vi "Read.vi"(8 "error in (no error)":errorcluster, 9 "Sample Rate [Hz]":dbl=1000.0 min=1000.0 max=1000000.0, 10 "Number of Samples":u32=1000, 11 "AI (N Samples) Ref In":T1) -> (0 "error out":errorcluster, 2 "Values":dbl[][](array[numeric]), 3 "AI (N Samples) Ref Out":T1)   [LabVIEW 2021, in "AI Block.lvlib"]
doc: "Reads values from one or more analog input channels. Use this VI to read multiple samples for each channel at one time."
uses:
  <vilib>/myRIO/Instrument Drivers/Onboard IO/AI Block/AI Block.lvlib
  <vilib>/myRIO/Instrument Drivers/Onboard IO/AI Block/typedefs/AI Block Reference.ctl
  <vilib>/myRIO/Common/Instrument Driver Framework/Utilities/typedefs/myRIO Generic Hardware Reference.ctl
  <vilib>/myRIO/Common/Instrument Driver Framework/Utilities/typedefs/Hardware Version Enum.ctl
  <vilib>/myRIO/Common/Instrument Driver Framework/Utilities/typedefs/myRIO v1.0 Reference.ctl
  <vilib>/myRIO/Common/Instrument Driver Framework/Utilities/typedefs/Generic FPGA Reference.ctl
  <vilib>/myRIO/Common/Instrument Driver Framework/myRIO v1.0/AI Block/typedefs/AI Block Channels List.ctl
  <vilib>/myRIO/Common/Instrument Driver Framework/myRIO v1.0/AI Block/typedefs/AI Block Channels Enum.ctl
  <vilib>/myRIO/Common/Instrument Driver Framework/Utilities/typedefs/Analog Scaling Constants.ctl
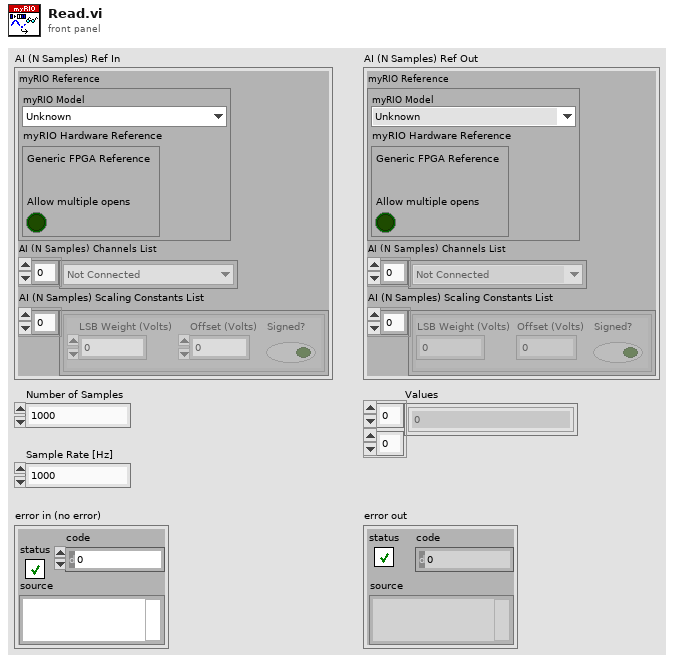
[diagram p1: front panel]
types:
  T1 = typedef "AI Block.lvlib/AI Block Reference.ctl" = cluster{"myRIO Reference":T2, "AI (N Samples) Channels List":T6, "AI (N Samples) Scaling Constants List":T8[]}
  T2 = typedef "myRIO Generic Hardware Reference.ctl" = cluster{"myRIO Model":T3, "myRIO Hardware Reference":T4}
  T3 = typedef "Hardware Version Enum.ctl" = enum16{"Unknown", "myRIO-1900", "myRIO-1950", "roboRIO", "NI ELVIS RIO CM", "ELVIS III"}
  T4 = typedef "myRIO v1.0 Reference.ctl" = cluster{"Generic FPGA Reference":T5, "Allow multiple opens":bool}
  T5 = typedef "Generic FPGA Reference.ctl" = refnum<k20>
  T6 = typedef "AI Block Channels List.ctl" = T7[]
  T7 = typedef "AI Block Channels Enum.ctl" = enum16{"Not Connected", "A/AI0 (N Samples)", "A/AI1 (N Samples)", "A/AI2 (N Samples)", "A/AI3 (N Samples)", "A/AI4 (N Samples)", "A/AI5 (N Samples)", "A/AI6 (N Samples)", "A/AI7 (N Samples)", "A/AI0 (DIFF N Samples)", "A/AI1 (DIFF N Samples)", "A/AI2 (DIFF N Samples)", "A/AI3 (DIFF N Samples)", "B/AI0 (N Samples)", "B/AI1 (N Samples)", "B/AI2 (N Samples)", "B/AI3 (N Samples)", "B/AI4 (N Samples)", "B/AI5 (N Samples)", "B/AI6 (N Samples)", "B/AI7 (N Samples)", "B/AI0 (DIFF N Samples)", "B/AI1 (DIFF N Samples)", "B/AI2 (DIFF N Samples)", "B/AI3 (DIFF N Samples)"}
  T8 = typedef "Analog Scaling Constants.ctl" = cluster{"LSB Weight (Volts)":dbl, "Offset (Volts)":dbl, "Signed?":bool}
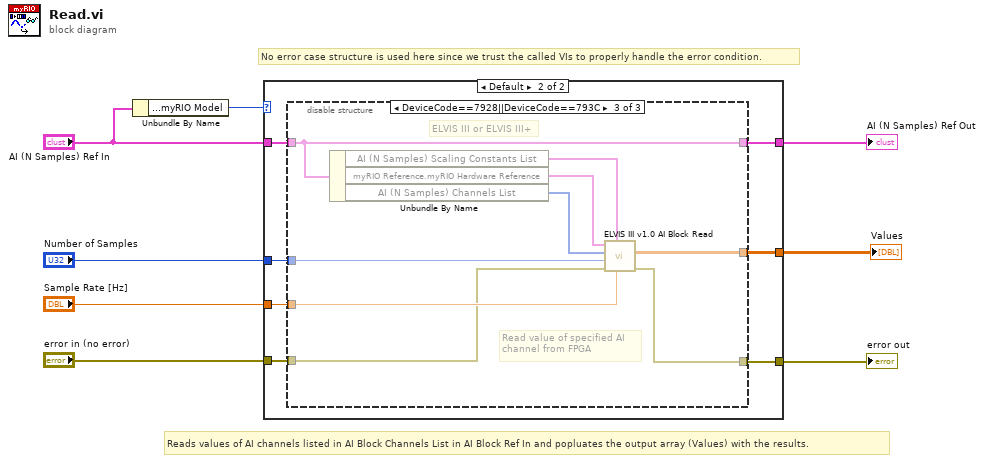
[diagram p0: block diagram]
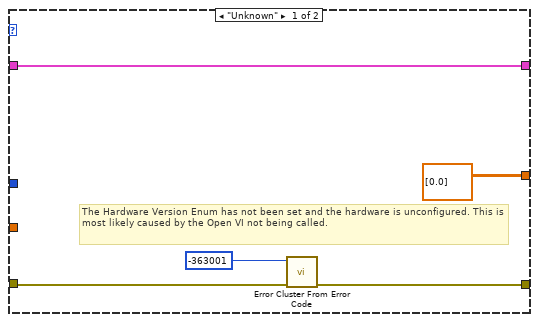
[diagram p2: hidden frame]
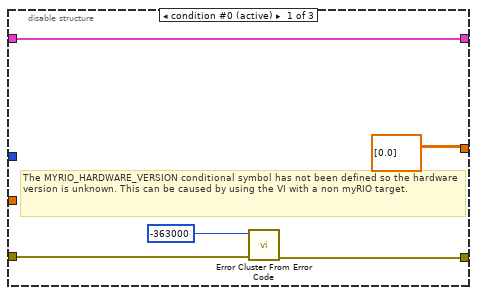
[diagram p3: hidden frame]
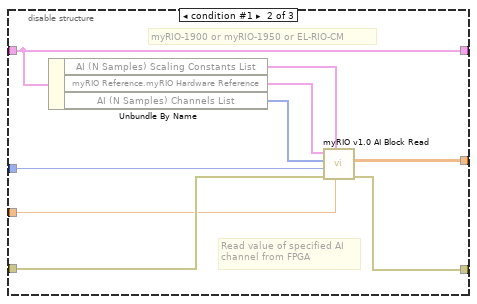
[diagram p4: hidden frame]
diagram:
  # "No error case structure is used here since we trust the called VIs to properly handle the error condition."
  # "Reads values of AI channels listed in AI Block Channels List in AI Block Ref In and popluates the output array (Values) with the results."
  n1 = Unbundle By Name("AI (N Samples) Ref In") -> ("myRIO Reference.myRIO Model"=w3:T3)
  n2 = case shown="Default" w3 {
    tunnel: [w11 w20] -> w5
    tunnel: "AI (N Samples) Ref In" -> [w10 w19]
    tunnel: "error in (no error)" -> [w12 w18]
    tunnel: [w10 w17] -> w6
    tunnel: [dbl[][] [[0.0]] w16] -> w4
    tunnel: "Sample Rate [Hz]" -> [_ w15]
    tunnel: "Number of Samples" -> [_ w14]
    frame "Unknown" {
      # "The Hardware Version Enum has not been set and the hardware is unconfigured. This is most likely caused by the Open VI not being called."
      n3 = call <vilib>:"Error Cluster From Error Code.vi"("error in (no error)"=w12, "error code (0)"=-363001) -> ("error out"=w11:errorcluster)  [unwired: 7 in]
    }
    frame Default {
      n4 = disable-structure shown="DeviceCode==7928||DeviceCode==793C" {
        disable-tunnel: w19 -> [w22 w27 w40]
        disable-tunnel: [w25 w33 w38] -> w20
        disable-tunnel: w18 -> [w23 w34 w35]
        disable-tunnel: [w22 w27 w40] -> w17
        disable-tunnel: [dbl[][] [[0.0]] ("dbl Scaled Value List") w31 w39] -> w16
        disable-tunnel: w15 -> [_ w28 w36]
        disable-tunnel: w14 -> [_ w30 w37]
        frame condition #0 (active) {
          # "The MYRIO_HARDWARE_VERSION conditional symbol has not been defined so the hardware version is unknown. This can be caused by using the VI with a non myRIO target."
          n5 = call <vilib>:"Error Cluster From Error Code.vi"("error in (no error)"=w23, "error code (0)"=-363000) -> ("error out"=w25:errorcluster)  [unwired: 7 in]
        }
        frame condition #1 {
          # "myRIO-1900 or myRIO-1950 or EL-RIO-CM"
          # "Read value of specified AI \nchannel from FPGA"
          n6 = Unbundle By Name(w27) -> ("AI (N Samples) Scaling Constants List"=w26:T8[], "myRIO Reference.myRIO Hardware Reference"=w32:T4, "AI (N Samples) Channels List"=w29:T6)
          n7 = call <vilib>:"myRIO v1.0 AI Block Read.vi"("AI FIFO Sample Rate"=w28, "Scale Constants Array"=w26, "error in (no error)"=w34, "Number of Samples"=w30, "AI (N Samples) Channels List"=w29, "myRIO Ref In"=w32) -> ("error out"=w33:errorcluster, "dbl Scaled Value List"=w31:dbl[][])  [unwired: 3 in, 1 out]
        }
        frame condition #2 {
          # "ELVIS III or ELVIS III+"
          # "Read value of specified AI \nchannel from FPGA"
          n8 = Unbundle By Name(w40) -> ("AI (N Samples) Scaling Constants List"=w41:T8[], "myRIO Reference.myRIO Hardware Reference"=w43:T4, "AI (N Samples) Channels List"=w42:T6)
          n9 = call <vilib>:"ELVIS III v1.0 AI Block Read.vi"("AI FIFO Sample Rate"=w36, "Scale Constants Array"=w41, "error in (no error)"=w35, "Number of Samples"=w37, "AI (N Samples) Channels List"=w42, "myRIO Ref In"=w43) -> ("error out"=w38:errorcluster, "dbl Scaled Value List"=w39:dbl[][])  [unwired: 3 in, 1 out]
        }
      }
    }
  }
  "AI (N Samples) Ref Out" <- w6
  "error out" <- w5
  "Values" <- w4
